vi "DamnYankeeHindbrainAct.vi"(10 "NotifierReff":T9, 11 "IO Port Cluster":T8) -> (0 "error out":errorcluster)   [LabVIEW 2013]
uses:
  Data/TypeDefs/Notifiers.ctl
  Data/TypeDefs/UTM Location.ctl
  Data/TypeDefs/Sail Set Suggestions.ctl
  Data/TypeDefs/Rudder Set Suggestions.ctl
  Data/TypeDefs/OverrideInformation.ctl
  Data/TypeDefs/OverrideMode.ctl
  Data/TypeDefs/MotorSetup.ctl
  Data/TypeDefs/DynamixelSetupInfo.ctl
  Data/TypeDefs/AirmarStatus.ctl
  <vilib>/myRIO/Instrument Drivers/Onboard IO/PWM/typedefs/PWM Reference.ctl
  <vilib>/myRIO/Common/Instrument Driver Framework/Utilities/typedefs/myRIO Generic Hardware Reference.ctl
  <vilib>/myRIO/Common/Instrument Driver Framework/Utilities/typedefs/Hardware Version Enum.ctl
  <vilib>/myRIO/Common/Instrument Driver Framework/Utilities/typedefs/myRIO v1.0 Reference.ctl
  <vilib>/myRIO/Common/Instrument Driver Framework/Utilities/typedefs/Generic FPGA Reference.ctl
  <vilib>/myRIO/Common/Instrument Driver Framework/myRIO v1.0/PWM/typedefs/PWM Channels Enum.ctl
  <vilib>/myRIO/Instrument Drivers/Onboard IO/PWM/typedefs/PWM Configuration.ctl
  <vilib>/myRIO/Instrument Drivers/Onboard IO/PWM/PWM.lvlib
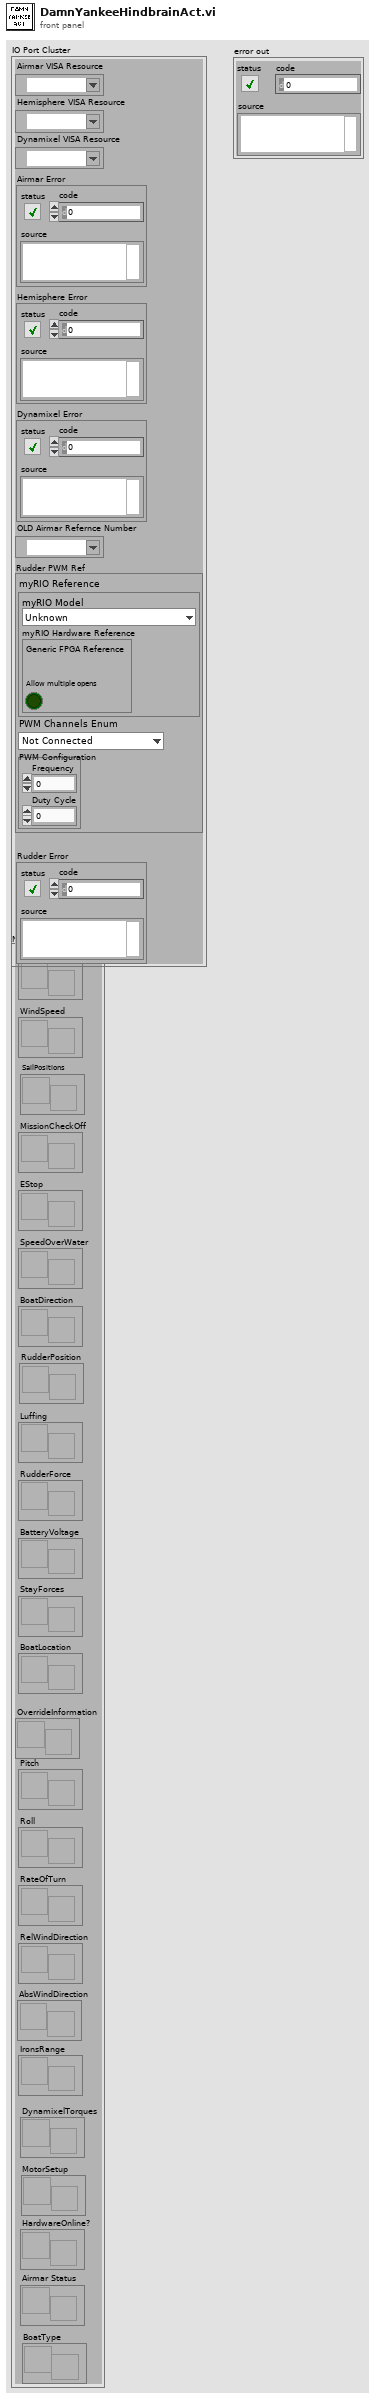
[diagram p1: front panel]
types:
  T1 = typedef "PWM.lvlib/PWM Reference.ctl" = cluster{"myRIO Reference":T2, "PWM Channels Enum":T6, "PWM Configuration":T7}
  T2 = typedef "myRIO Generic Hardware Reference.ctl" = cluster{"myRIO Model":T3, "myRIO Hardware Reference":T4}
  T3 = typedef "Hardware Version Enum.ctl" = enum16{"Unknown", "myRIO-1900", "myRIO-1950"}
  T4 = typedef "myRIO v1.0 Reference.ctl" = cluster{"Generic FPGA Reference":T5, "Allow multiple opens":bool}
  T5 = typedef "Generic FPGA Reference.ctl" = refnum<k20>
  T6 = typedef "PWM Channels Enum.ctl" = enum16{"Not Connected", "C/PWM0", "C/PWM1", "A/PWM0", "A/PWM1", "A/PWM2", "B/PWM0", "B/PWM1", "B/PWM2"}
  T7 = typedef "PWM.lvlib/PWM Configuration.ctl" = cluster{"Frequency":dbl, "Duty Cycle":dbl}
  T8 = cluster{"Airmar VISA Resource":refnum<visa-resource-name>, "Hemisphere VISA Resource":refnum<visa-resource-name>, "Dynamixel VISA Resource":refnum<visa-resource-name>, "Airmar Error":errorcluster, "Hemisphere Error":errorcluster, "Dynamixel Error":errorcluster, "OLD Airmar Refernce Number":refnum<visa-resource-name>, "Rudder PWM Ref":T1, "Rudder Error":errorcluster}
  T9 = typedef "Notifiers.ctl" = cluster{"BoatSpeed":refnum<notifier>, "WindSpeed":refnum<notifier>, "MissionCheckOff":refnum<notifier>, "EStop":refnum<notifier>, "SpeedOverWater":refnum<notifier>, "BoatDirection":refnum<notifier>, "Luffing":refnum<notifier>, "RudderForce":refnum<notifier>, "BatteryVoltage":refnum<notifier>, "StayForces":refnum<notifier>, "BoatLocation":refnum<notifier>, "Pitch":refnum<notifier>, "Roll":refnum<notifier>, "RateOfTurn":refnum<notifier>, "RelWindDirection":refnum<notifier>, "SailPositions":refnum<notifier>, "RudderPosition":refnum<notifier>, "IronsRange":refnum<notifier>, "AbsWindDirection":refnum<notifier>, "OverrideInformation":refnum<notifier>, "DynamixelTorques":refnum<notifier>, "HardwareOnline?":refnum<notifier>, "MotorSetup":refnum<notifier>, "Airmar Status":refnum<notifier>, "BoatType":refnum<notifier>}
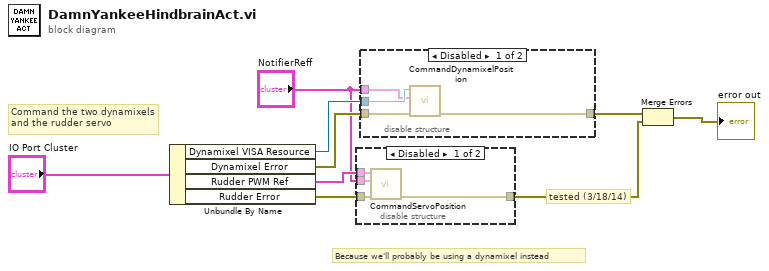
[diagram p0: block diagram]
diagram:
  # "Because we'll probably be using a dynamixel instead"
  # "tested (3/18/14)"
  # "Command the two dynamixels and the rudder servo"
  n1 = Unbundle By Name("IO Port Cluster") -> ("Dynamixel VISA Resource"=w6:refnum<visa-resource-name>, "Dynamixel Error"=w7:errorcluster, "Rudder PWM Ref"=w8:T1, "Rudder Error"=w9:errorcluster)
  n2 = disable-structure shown="Disabled" {
    disable-tunnel: w9 -> [w13 _]
    disable-tunnel: w8 -> [w12 _]
    disable-tunnel: [w11 _] -> w2
    disable-tunnel: "NotifierReff" -> [w10 _]
    frame Disabled {
      n3 = call "CommandServoPosition.vi"("PWM Ref In"=w12, "NotifierReff"=w10, "Error in"=w13) -> ("Error out"=w11:errorcluster)  [unwired: 7 in]
    }
    frame Enabled {
    }
  }
  n4 = disable-structure shown="Disabled" {
    disable-tunnel: [w17 _] -> w4
    disable-tunnel: w6 -> [w16 _]
    disable-tunnel: w7 -> [w15 _]
    disable-tunnel: "NotifierReff" -> [w14 _]
    frame Disabled {
      n5 = call "CommandDynamixelPosition.vi"("Error in"=w15, "NotifierReff"=w14, "VISA resource name"=w16) -> ("Error out"=w17:errorcluster)  [unwired: 8 in]
    }
    frame Enabled {
    }
  }
  n6 = Merge Errors "Merge Errors"(w4, w2) -> (→"error out":errorcluster)
